vi "VirtualDice.vi"() -> ()   [LabVIEW 2021]
panel:
  in  "stop":bool
  in  "Numeric":dbl
  out "A6":bool
  out "A3":bool
  out "A5":bool
  out "A4":bool
  out "A7":bool
  out "A2":bool
  out "A1":bool
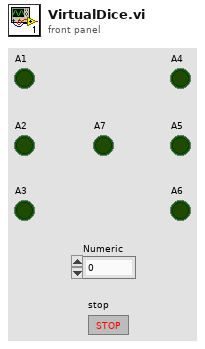
[diagram p1: front panel]
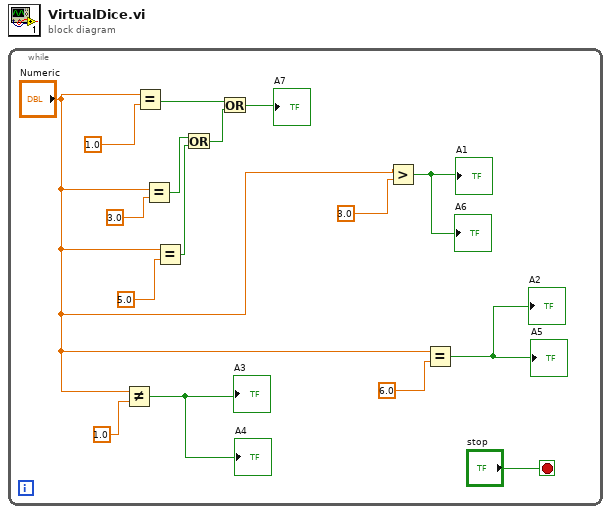
[diagram p0: block diagram]
diagram:
  n1 = while {
    stop <- "stop" stop-if-true
    n2 = Not Equal?(x="Numeric", y=1.0 ("Numeric")) -> (x != y?=→"A4" →"A3":bool)
    n3 = Equal?(x="Numeric", y=1.0 ("Numeric")) -> (x = y?=w3:bool)
    n4 = Equal?(x="Numeric", y=3.0 ("Numeric")) -> (x = y?=w4:bool)
    n5 = Equal?(x="Numeric", y=5.0 ("Numeric")) -> (x = y?=w14:bool)
    n6 = Or(x=w4, y=w14) -> (x .or. y?=w16:bool)
    n7 = Or(x=w3, y=w16) -> (x .or. y?=→"A7":bool)
    n8 = Greater?(x="Numeric", y=3.0 ("Numeric")) -> (0:→"A1" →"A6":bool)
    n9 = Equal?(x="Numeric", y=6.0 ("Numeric")) -> (x = y?=→"A2" →"A5":bool)
  }
